vi "Destroy.vi"(0 "reference":refnum<class "LineStyle.lvclass">, 5 "error in (no error)":errorcluster) -> (19 "error out":errorcluster)   [LabVIEW 2016, in "LineStyle.lvclass"]
doc: "Destroys an object created with a LineStyle constructor VI or a subclass of the LineStyle class. This VI must be reentrant.\n\n[GOOP 2.1]"
uses:
  <resource>/Framework/Providers/Open_GDS/UML/LineStyle_class/LineStyle.lvclass
panel:
  out "reference out":refnum<class "LineStyle.lvclass">
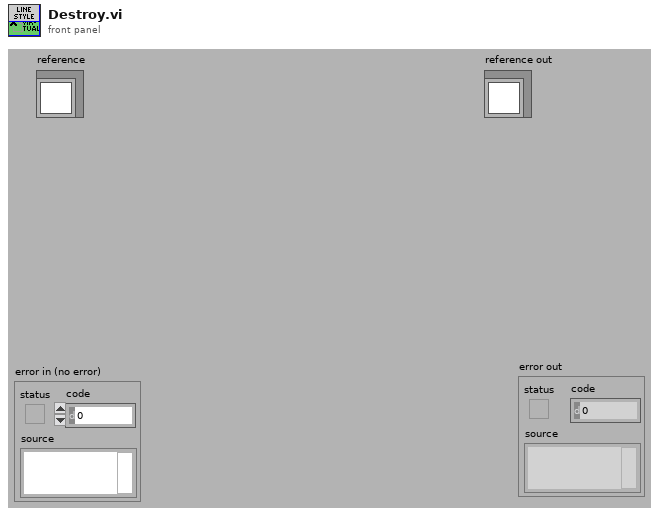
[diagram p1: front panel]
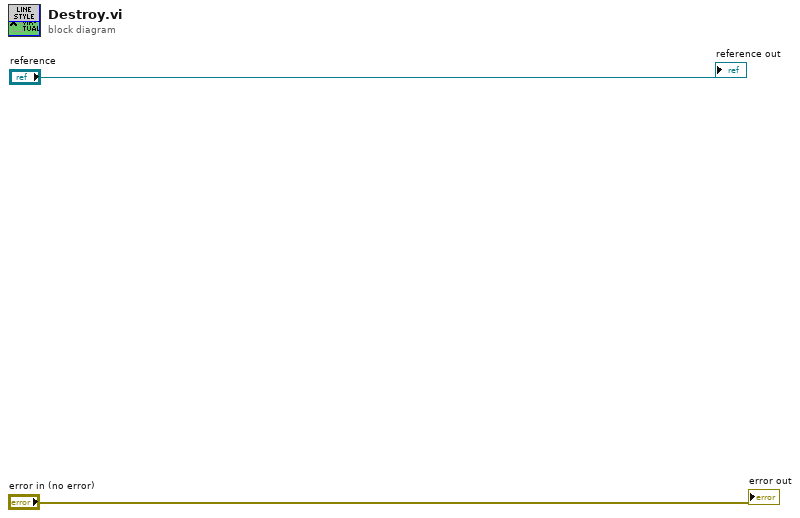
[diagram p0: block diagram]
diagram:
  "error out" <- "error in (no error)"
  "reference out" <- "reference"
